vi "CRIO_String2State.vi"(8 "error in (no error)":errorcluster, 10 "Curr State":T1, 11 "data in":string) -> (0 "error out":errorcluster, 3 "Command State":T1)   [LabVIEW 2017]
uses:
  CRIO_StateEnum.ctl
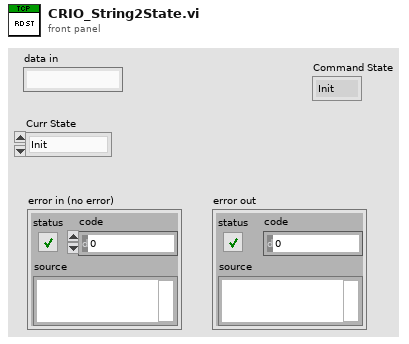
[diagram p1: front panel]
types:
  T1 = typedef "CRIO_StateEnum.ctl" = enum16{"Init", "Listen", "Wait", "Setup", "Ready to Launch", "Start Flight", "Accelerating", "Coasting", "Braking", "End Flight", "Loading", "Stop"}
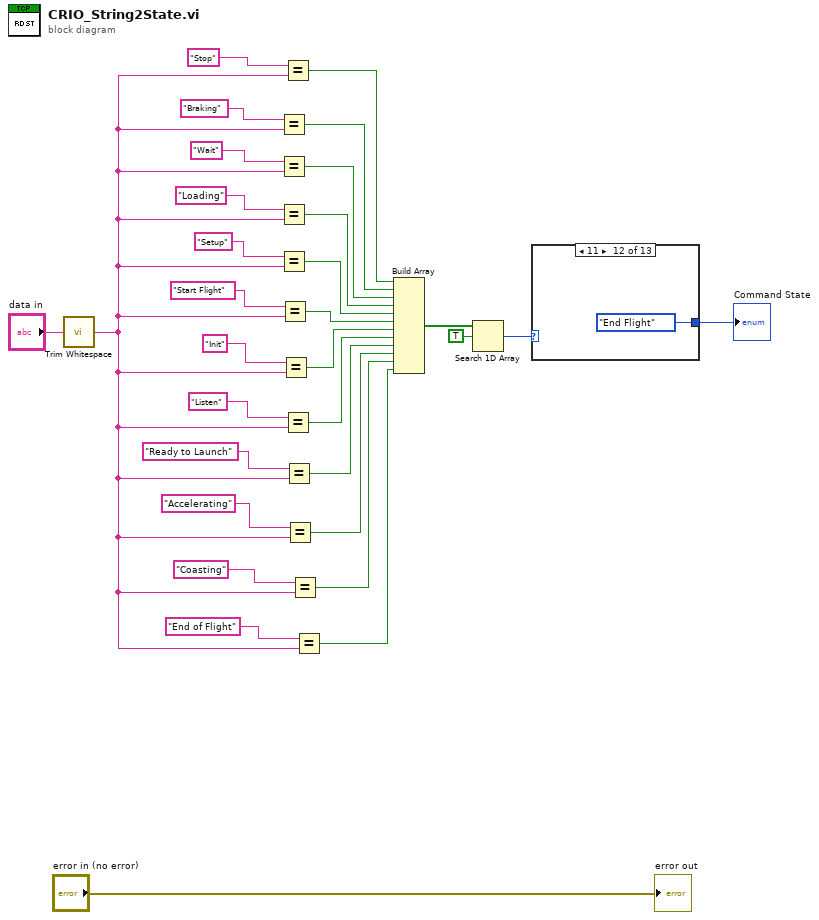
[diagram p0: block diagram]
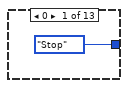
[diagram p2: hidden frame]
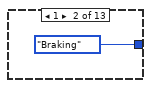
[diagram p3: hidden frame]
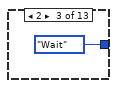
[diagram p4: hidden frame]
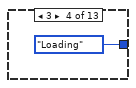
[diagram p5: hidden frame]
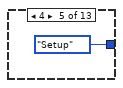
[diagram p6: hidden frame]
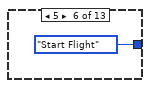
[diagram p7: hidden frame]
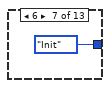
[diagram p8: hidden frame]
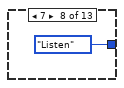
[diagram p9: hidden frame]
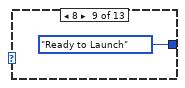
[diagram p10: hidden frame]
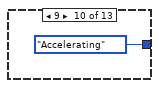
[diagram p11: hidden frame]
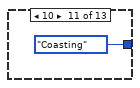
[diagram p12: hidden frame]
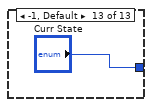
[diagram p13: hidden frame]
diagram:
  n1 = call <vilib>:"Trim Whitespace.vi"("string"="data in") -> ("trimmed string"=w2:string)  [unwired: 1 in]
  n2 = Equal?(x="Braking" ("y"), y=w2) -> (x = y?=w29:bool)
  n3 = Equal?(x="Wait" ("y"), y=w2) -> (x = y?=w25:bool)
  n4 = Equal?(x="Loading" ("y"), y=w2) -> (x = y?=w24:bool)
  n5 = Equal?(x="Setup" ("y"), y=w2) -> (x = y?=w23:bool)
  n6 = Equal?(x="Start Flight" ("y"), y=w2) -> (x = y?=w15:bool)
  n7 = Equal?(x="Init" ("y"), y=w2) -> (x = y?=w8:bool)
  n8 = Equal?(x="Stop" ("y"), y=w2) -> (x = y?=w17:bool)
  n9 = Equal?(x="Listen" ("y"), y=w2) -> (x = y?=w7:bool)
  n10 = Equal?(x="Ready to Launch" ("y"), y=w2) -> (x = y?=w6:bool)
  n11 = Equal?(x="Accelerating" ("y"), y=w2) -> (x = y?=w5:bool)
  n12 = Equal?(x="Coasting" ("y"), y=w2) -> (x = y?=w4:bool)
  n13 = Equal?(x="End of Flight" ("y"), y=w2) -> (x = y?=w1:bool)
  n14 = Build Array(w17, w29, w25, w24, w23, w15, w8, w7, w6, w5, w4, w1) -> (w21:bool[])
  n15 = Search 1D Array(1D array=w21, element=TRUE) -> (index of element=w20:i32)  [unwired: 1 in]
  n16 = case shown="11" w20 {
    tunnel: [CRIO_StateEnum."Stop" ("States") CRIO_StateEnum."Braking" ("States") CRIO_StateEnum."Wait" ("States") CRIO_StateEnum."Loading" ("States") CRIO_StateEnum."Setup" ("States") CRIO_StateEnum."Start Flight" ("States") CRIO_StateEnum."Init" ("States") CRIO_StateEnum."Listen" ("States") CRIO_StateEnum."Ready to Launch" ("States") CRIO_StateEnum."Accelerating" ("States") CRIO_StateEnum."Coasting" ("States") CRIO_StateEnum."End Flight" ("States") "Curr State"] -> w19
    frame 0 {
    }
    frame 1 {
    }
    frame 2 {
    }
    frame 3 {
    }
    frame 4 {
    }
    frame 5 {
    }
    frame 6 {
    }
    frame 7 {
    }
    frame 8 {
    }
    frame 9 {
    }
    frame 10 {
    }
    frame 11 {
    }
    frame -1, Default {
    }
  }
  "Command State" <- w19
  "error out" <- "error in (no error)"
